vi "test variant to json float.vi"(8 "error in (no error)":errorcluster) -> (0 "error out":errorcluster)   [LabVIEW 2019, in "labview_json_tests.lvlib"]
uses:
  labview_json_tests.lvlib
  lib/labview_json.lvlib
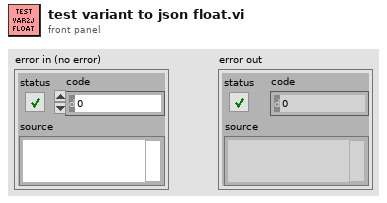
[diagram p1: front panel]
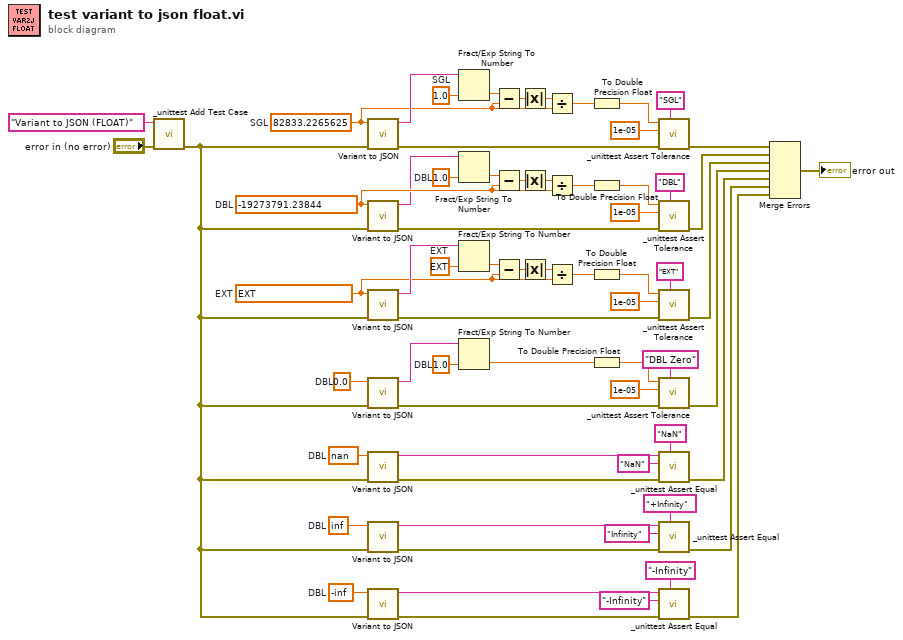
[diagram p0: block diagram]
diagram:
  w7 = -inf  # DBL
  w9 = inf  # DBL
  w19 = nan  # DBL
  w27 = 1.0  # DBL
  w20 = 0.0  # DBL
  w39 = ext 1.0  # EXT
  w35 = ext 12803819273791.238  # EXT
  w43 = 1.0  # DBL
  w47 = -19273791.23844  # DBL
  w63 = sgl 1.0  # SGL
  w59 = sgl 82833.23  # SGL
  n1 = call "_unittest Add Test Case.vi"("error in (no error)"="error in (no error)", "Test Case"="Variant to JSON (FLOAT)") -> ("error out"=w1:errorcluster)  [unwired: 9 in]
  n2 = call "Variant to JSON.vi"("error in (no error)"=w1, "Variant in"=w59) -> ("error out"=w58:errorcluster, "JSON"=w64:string)  [unwired: 8 in]
  n3 = call "Variant to JSON.vi"("error in (no error)"=w1, "Variant in"=w47) -> ("error out"=w48:errorcluster, "JSON"=w42:string)  [unwired: 8 in]
  n4 = call "Variant to JSON.vi"("error in (no error)"=w1, "Variant in"=w35) -> ("error out"=w34:errorcluster, "JSON"=w40:string)  [unwired: 8 in]
  n5 = call "Variant to JSON.vi"("error in (no error)"=w1, "Variant in"=w20) -> ("error out"=w26:errorcluster, "JSON"=w28:string)  [unwired: 8 in]
  n6 = call "Variant to JSON.vi"("error in (no error)"=w1, "Variant in"=w19) -> ("error out"=w18:errorcluster, "JSON"=w17:string)  [unwired: 8 in]
  n7 = call "Variant to JSON.vi"("error in (no error)"=w1, "Variant in"=w9) -> ("error out"=w10:errorcluster, "JSON"=w11:string)  [unwired: 8 in]
  n8 = call "Variant to JSON.vi"("error in (no error)"=w1, "Variant in"=w7) -> ("error out"=w6:errorcluster, "JSON"=w5:string)  [unwired: 8 in]
  n9 = Fract/Exp String To Number(string=w64, default (0 dbl)=w63) -> (number=w60:sgl)  [unwired: 2 in, 1 out]
  n10 = Fract/Exp String To Number(string=w42, default (0 dbl)=w43) -> (number=w46:dbl)  [unwired: 2 in, 1 out]
  n11 = Fract/Exp String To Number(string=w40, default (0 dbl)=w39) -> (number=w36:ext)  [unwired: 2 in, 1 out]
  n12 = Fract/Exp String To Number(string=w28, default (0 dbl)=w27) -> (number=w21:dbl)  [unwired: 2 in, 1 out]
  n13 = Subtract(x=w60, y=w59) -> (x-y=w62:sgl)
  n14 = Subtract(x=w46, y=w47) -> (x-y=w44:dbl)
  n15 = Subtract(x=w36, y=w35) -> (x-y=w38:ext)
  n16 = Absolute Value(x=w62) -> (abs(x)=w61:sgl)
  n17 = Absolute Value(x=w44) -> (abs(x)=w45:dbl)
  n18 = Absolute Value(x=w38) -> (abs(x)=w37:ext)
  n19 = Divide(x=w61, y=w59) -> (x/y=w55:sgl)
  n20 = Divide(x=w45, y=w47) -> (x/y=w50:dbl)
  n21 = Divide(x=w37, y=w35) -> (x/y=w32:ext)
  n22 = To Double Precision Float(number=w55) -> (double precision float=w54:dbl)
  n23 = To Double Precision Float(number=w50) -> (double precision float=w51:dbl)
  n24 = To Double Precision Float(number=w32) -> (double precision float=w31:dbl)
  n25 = To Double Precision Float(number=w21) -> (double precision float=w24:dbl)
  n26 = call "_unittest Assert Tolerance.vi"("Message"="SGL", "error in (no error)"=w58, "Tollerance (1E-5)"=1e-05, "Actual Value"=w54) -> ("error out"=w57:errorcluster)  [unwired: 7 in]
  n27 = call "_unittest Assert Tolerance.vi"("Message"="DBL", "error in (no error)"=w48, "Tollerance (1E-5)"=1e-05, "Actual Value"=w51) -> ("error out"=w41:errorcluster)  [unwired: 7 in]
  n28 = call "_unittest Assert Tolerance.vi"("Message"="EXT", "error in (no error)"=w34, "Tollerance (1E-5)"=1e-05, "Actual Value"=w31) -> ("error out"=w29:errorcluster)  [unwired: 7 in]
  n29 = call "_unittest Assert Tolerance.vi"("Message"="DBL Zero", "error in (no error)"=w26, "Tollerance (1E-5)"=1e-05, "Actual Value"=w24) -> ("error out"=w22:errorcluster)  [unwired: 7 in]
  n30 = call "_unittest Assert Equal.vi"("Message"="NaN", "error in (no error)"=w18, "Expected Value"="NaN", "Actual Value"=w17) -> ("error out"=w16:errorcluster)  [unwired: 7 in]
  n31 = call "_unittest Assert Equal.vi"("Message"="+Infinity", "error in (no error)"=w10, "Expected Value"="Infinity", "Actual Value"=w11) -> ("error out"=w8:errorcluster)  [unwired: 7 in]
  n32 = call "_unittest Assert Equal.vi"("Message"="-Infinity", "error in (no error)"=w6, "Expected Value"="-Infinity", "Actual Value"=w5) -> ("error out"=w2:errorcluster)  [unwired: 7 in]
  n33 = Merge Errors(w57, w41, w29, w22, w16, w8, w2) -> (→"error out":errorcluster)
